vi "Actor Core.vi"(8 "error in":errorcluster, 11 "Manual Control in":refnum<class "Manual Control.lvclass">) -> (0 "error out":errorcluster, 3 "Actor out":refnum<class "Actor.lvclass">)   [LabVIEW 2018, in "Manual Control Actor.lvlib" / "Manual Control.lvclass"]
doc: "(<B>Filename</B>: Actor Framework.lvlib:Actor.lvclass:Actor Core.vi)\n\nReceives messages to the actor, reacts to them, and initiates any error handling that may shut the actor down.\n\nDescendant classes may override this VI to append parallel tasks for the actor to complete while it handles messages. Overrides use the Call Parent Method node."
uses:
  Manual Control.lvclass
  C:/Users/Administrator/Desktop/2018LabVIEW EMS/EMS Generic Actor/EMS Generic/EMS Generic.lvclass
  C:/Program Files (x86)/National Instruments/LabVIEW 2018/vi.lib/ActorFramework/Actor/Actor.lvclass
  C:/Users/Administrator/Desktop/2018LabVIEW EMS/Device Communication and Control Abstract Actor/Device Communication and Control Abstract/Device Communication and Control Abstract.lvclass
  <vilib>/ActorFramework/Actor/Actor.lvclass
  EMS Generic Actor/EMS Generic/EMS Generic.lvclass/EMS Generic.ctl
  Manual Control.lvclass/Manual Control.ctl
  <vilib>/ActorFramework/Actor/Actor.lvclass/Actor.ctl
  Device Communication and Control Abstract Actor/Device Communication and Control Abstract/Device Communication and Control Abstract.lvclass/Device Communication and Control Abstract.ctl
  <vilib>/ActorFramework/Message Enqueuer/Message Enqueuer.lvclass/Message Enqueuer.ctl
  EMS Generic Actor/EMS Generic Messages/Return DER_Measurement Msg/Return DER_Measurement Msg.lvclass/Return DER_Measurement Msg.ctl
  <vilib>/ActorFramework/Message Enqueuer/Enqueue.vi
  EMS Generic Actor/EMS Generic/Accessors - Abstract Messages/Read Return DER_Measurement Msg.vi
  EMS Generic Actor/EMS Generic Messages/Return DER_Measurement Msg/Send Return DER_Measurement.vi
  Device Communication and Control Abstract Actor/Device Communication and Control Abstract Messages/Set IED MicrogridID Msg/Set IED MicrogridID Msg.lvclass
  C:/Program Files (x86)/National Instruments/LabVIEW 2018/vi.lib/ActorFramework/Message/Message.lvclass
  EMS Generic Actor/EMS Generic Messages/Return DER_Measurement Msg/Return DER_Measurement Msg.lvclass
  <vilib>/ActorFramework/Message Priority Queue/Priority Enqueue.vi
  Utilities/Determine Device Types.vi
  EMS Generic Actor/EMS Generic/DVR Readers/Read Smart Relay Measurement DVR.vi
  EMS Generic Actor/EMS Generic/DVR Readers/Read DER Measurement DVR.vi
  Generic Optimization Actor/Generic Optimization/Generic Optimization.lvclass
  EMS Generic Actor/EMS Generic/EMS Generic.lvclass
  Device Communication and Control Abstract Actor/Device Communication and Control Abstract/Device Communication and Control Abstract.lvclass
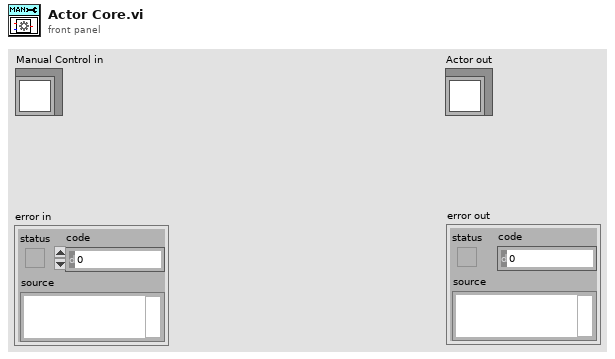
[diagram p1: front panel]
types:
  T1 = typedef "EMS Generic Actor.lvlib/EMS Generic.lvclass/Data Type DVRs.ctl" = cluster{"IED_Status":refnum<data-value>, "IED_Status_0":refnum<data-value>, "DER_Measurement":refnum<data-value>, "DER_Info":refnum<data-value>, "DER_Status":refnum<data-value>, "ES_Measurement":refnum<data-value>, "ES_Info":refnum<data-value>, "PV_Info":refnum<data-value>, "SmartRelay_Info":refnum<data-value>, "SmartRelay_Measurement":refnum<data-value>, "Meter_Info":refnum<data-value>, "Meter_Measurement":refnum<data-value>, "HVAC_Status":refnum<data-value>, "HVAC_Measurement":refnum<data-value>, "PriceData_RealTime":refnum<data-value>, "PriceData_Demand":refnum<data-value>, "PriceData_Energy":refnum<data-value>, "ForecastData_Long":refnum<data-value>, "ForecastData_Short":refnum<data-value>, "DER_Control":refnum<data-value>, "DER_SetPointF":refnum<data-value>, "DER_SetPointP":refnum<data-value>, "DER_SetPointQ":refnum<data-value>, "DER_SetPointPF":refnum<data-value>, "DER_SetPointV":refnum<data-value>, "PV_setCurtailment":refnum<data-value>, "PV_setRampRate":refnum<data-value>, "Relay_Control":refnum<data-value>, "Load_Control":refnum<data-value>, "HVAC_Control":refnum<data-value>, "Generator_Info":refnum<data-value>, "ForecastData_Long_Backup":refnum<data-value>, "PriceData_RealTime_Backup":refnum<data-value>}
  T2 = typedef "CSEISMIC DDS.lvlib/CSEISMIC DDS.lvclass/DeviceID.ctl" = string
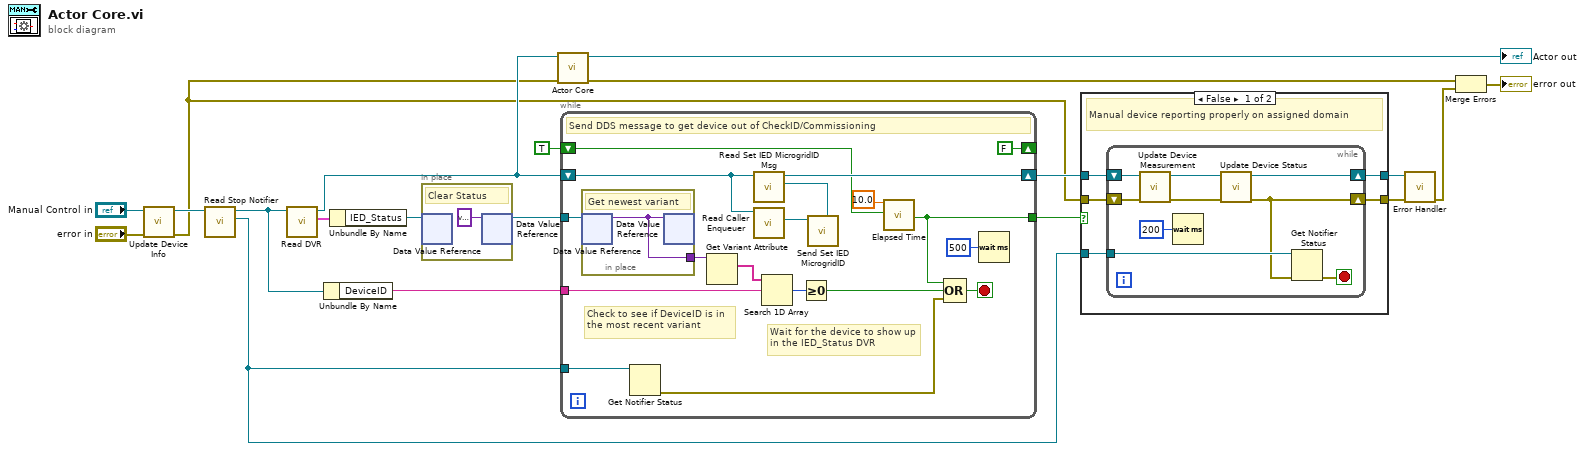
[diagram p0: block diagram]
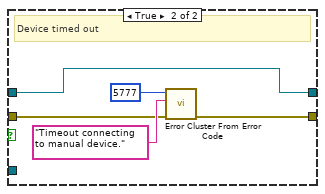
[diagram p2: hidden frame]
diagram:
  n1 = call "Update Device Info.vi"("error in"="error in", "Manual Control in"="Manual Control in") -> ("error out"=w2:errorcluster, "Manual Control out"=w9:refnum<class "Manual Control.lvclass">)  [unwired: 8 in]
  n2 = call "Read Stop Notifier.vi"("EMS Generic in"=w9) -> ("stop"=w12:refnum<notifier>, "EMS Generic out"=w8:refnum<class "Manual Control.lvclass">)  [unwired: 9 in]
  n3 = call "Read DVR.vi"("EMS Generic in"=w8) -> ("DVR"=w15:T1, "EMS Generic out"=w6:refnum<class "Manual Control.lvclass">)  [unwired: 9 in]
  n4 = Unbundle By Name(w8) -> ("DeviceID"=w13:T2)
  n5 = Unbundle By Name(w15) -> ("IED_Status"=w16:refnum<data-value>)
  n6 = in-place {
    # "Clear Status"
    n7 = in-place-dvr #1(w16) -> ()  [unwired: 2 out]
    n8 = in-place-dvr #1(variant ("data value")) -> (w14:refnum<data-value>)  [unwired: 1 out]
  }
  n9 = call-parent "Actor Core.vi"("error in"=w2, "Actor in"=w6) -> ("error out"=w5:errorcluster, "Actor out"=→"Actor out":refnum<class "Actor.lvclass">)  [unwired: 8 in]
  n10 = while {
    tunnel: w14 -> [w34]
    shift-right: [w35] -> w7
    shift-left: w6 -> [w36]
    tunnel: w13 -> [w30]
    tunnel: w12 -> [w28]
    tunnel: [w24] -> w11
    shift-right: [FALSE] -> _
    shift-left: TRUE -> [w23]
    stop <- w25 stop-if-true
    # "Check to see if DeviceID is in the most recent variant"
    # "Wait for the device to show up in the IED_Status DVR"
    # "Send DDS message to get device out of CheckID/Commissioning"
    n11 = in-place {
      in-place-border: [w40] -> w39
      # "Get newest variant"
      n12 = in-place-dvr #2(w34) -> (w40:variant)  [unwired: 1 out]
      n13 = in-place-dvr #2(w40) -> ()  [unwired: 2 out]
    }
    n14 = Get Notifier Status(notifier=w28) -> (error out=w26:errorcluster)  [unwired: 1 in, 4 out]
    n15 = Get Variant Attribute(Variant=w39) -> (names=w31:string[])  [unwired: 3 in, 3 out]
    n16 = call "Read Set IED MicrogridID Msg.vi"("SCADA Sub Abstract in"=w36) -> ("Set IED MicrogridID Msg"=w38:refnum<class "Set IED MicrogridID Msg.lvclass">, "SCADA Sub Abstract out"=w35:refnum<class "Manual Control.lvclass">)  [unwired: 9 in]
    n17 = call <vilib>:"Read Caller Enqueuer.vi"("Actor"=w36) -> ("Caller Enqueuer"=w37:refnum<class "Message Enqueuer.lvclass">)  [unwired: 10 in]
    n18 = Search 1D Array(1D array=w31, element=w30) -> (index of element=w29:i32)  [unwired: 1 in]
    n19 = Greater Or Equal To 0?(x=w29) -> (x >= 0?=w27:bool)
    n20 = call "Send Set IED MicrogridID.vi"("Message Type"=w38, "Message Enqueuer"=w37) -> ()  [unwired: 8 in, 2 out]
    n21 = call "Elapsed Time"("Time Target (s)"=10.0, "Reset"=w23) -> ("Time has Elapsed"=w24:bool)  [unwired: 10 in, 7 out]
    n22 = Compound Arithmetic op=OR(w24, w27, w26) -> (w25:bool)
    n23 = Wait (ms)(milliseconds to wait=u32 500) -> ()  [unwired: 1 out]
  }
  n24 = case shown="False" w11 {
    tunnel: w7 -> [w45 w59]
    tunnel: w2 -> [w44 w56]
    tunnel: [w43 w55] -> w18
    tunnel: [w42 w59] -> w17
    tunnel: w12 -> [w41 _]
    frame False {
      # "Manual device reporting properly on assigned domain"
      n25 = while {
        tunnel: w41 -> [w54]
        shift-right: [w48] -> w43
        shift-left: w44 -> [w51]
        shift-right: [w46] -> w42
        shift-left: w45 -> [w52]
        stop <- w53 stop-if-true
        n26 = call "Update Device Measurement.vi"("error in"=w51, "Manual Control in"=w52) -> ("error out"=w49:errorcluster, "Manual Control out"=w50:refnum<class "Manual Control.lvclass">)  [unwired: 8 in]
        n27 = Wait (ms)(milliseconds to wait=u32 200) -> ()  [unwired: 1 out]
        n28 = call "Update Device Status.vi"("error in"=w49, "Manual Control in"=w50) -> ("error out"=w48:errorcluster, "Manual Control out"=w46:refnum<class "Manual Control.lvclass">)  [unwired: 8 in]
        n29 = Get Notifier Status(notifier=w54, error in (no error)=w48) -> (error out=w53:errorcluster)  [unwired: 4 out]
      }
    }
    frame True {
      # "Device timed out"
      n30 = call <vilib>:"Error Cluster From Error Code.vi"("error in (no error)"=w56, "error message (\"\")"="Timeout connecting to manual device." ("error message (\"\")"), "error code (0)"=5777) -> ("error out"=w55:errorcluster)  [unwired: 6 in]
    }
  }
  n31 = call-dynamic "Error Handler.vi"("error in"=w18, "EMS Generic in"=w17) -> ("error out"=w4:errorcluster)  [unwired: 8 in, 1 out]
  n32 = Merge Errors(w5, w4) -> (→"error out":errorcluster)
